vi "ReadHeaterSettings.vi"(7 "Prepended command":string, 8 "error in (no error)":errorcluster, 11 "VISA Refnum in":refnum<visa-resource-name>) -> (0 "error out":errorcluster, 2 "Settings array out":dbl[](array[numeric]), 3 "VISA Refnum out":refnum<visa-resource-name>)   [LabVIEW 2017, in "Fridge Software v2.1.lvlib"]
uses:
  Fridge Software v2.1.lvlib
  <instrlib>/Lake Shore 372/Lake Shore 372.lvlib
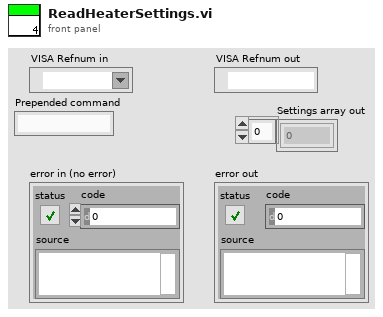
[diagram p1: front panel]
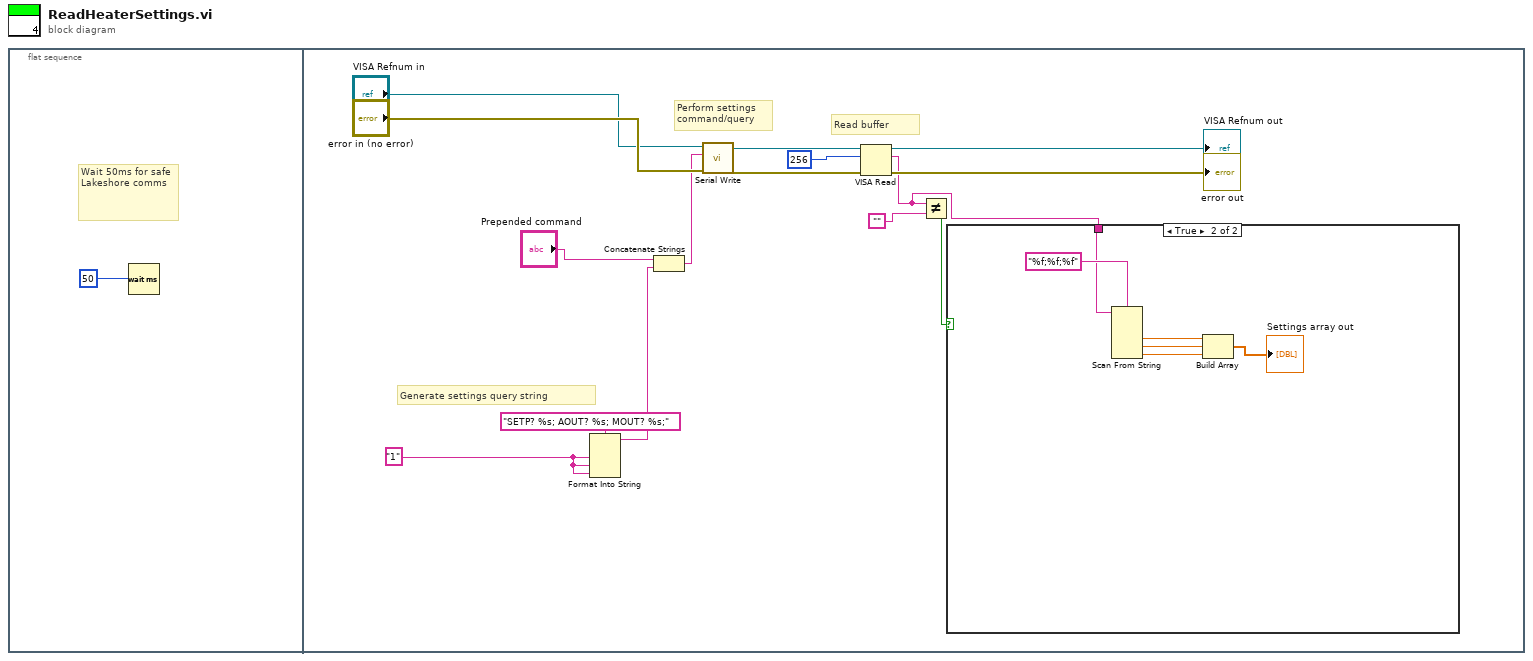
[diagram p0: block diagram]
diagram:
  n1 = flat-sequence {
    frame #0 {
      # "Wait 50ms for safe Lakeshore comms"
      n2 = Wait (ms)(milliseconds to wait=50) -> ()  [unwired: 1 out]
    }
    frame #1 {
      w2 = "1"
      # "Generate settings query string"
      # "Read buffer"
      # "Perform settings command/query"
      n3 = Format Into String(format string="SETP? %s; AOUT? %s; MOUT? %s;", w2, w2, w2) -> (resulting string=w7:string)  [unwired: 2 in, 1 out]
      n4 = Concatenate Strings("Prepended command", w7) -> (w6:string)
      n5 = call <instrlib>:"Serial Write.vi"("error in (no error)"="error in (no error)", "Write Buffer (\"\")"=w6, "VISA resource name"="VISA Refnum in") -> ("error out"=w12:errorcluster, "VISA resource name out"=w11:refnum<visa-resource-name>)  [unwired: 6 in, 1 out]
      n6 = VISA Read(VISA resource name=w11, byte count=u32 256, error in (no error)=w12) -> (VISA resource name out=→"VISA Refnum out":refnum<visa-resource-name>, read buffer=w3:string, error out=→"error out":errorcluster)  [unwired: 1 out]
      n7 = Not Equal?(x=w3, y="") -> (x != y?=w4:bool)
      n8 = case shown="True" w4 {
        tunnel: w3 -> [_ w19]
        frame False {
        }
        frame True {
          n9 = Scan From String(format string="%f;%f;%f", input string=w19) -> (output 1=w21:dbl, output 2=w22:dbl, output 3=w17:dbl)  [unwired: 5 in, 3 out]
          n10 = Build Array(w21, w22, w17) -> (→"Settings array out":dbl[])
        }
      }
    }
  }
